vi "Convert Detection Robot to AI Robot.vi"(7 "Lado":enum16{"Esquerdo", "Direito"}(ring) caption="Enum", 11 "Input":T6[](array[typedef]) {"height" format="%+4.3f"; "pixel_y" format="%+4.3f"; "pixel_x" format="%+4.3f"; "orientation" format="%+4.3f"; "y" format="%+4.3f"; "confidence" format="%4.3f"; "x" format="%+4.3f"}) -> (3 "Output":T1[](array[typedef]))   [LabVIEW 2018]
uses:
  Controls/SSL Detection Robot.ctl
  <vilib>/Analysis/Matrix/Datatypes/RealMatrix.ctl
  Communication_class/Paths/Convert AI Robot to Robot Command Folder/Core/AI Robot.ctl
  Communication_class/Paths/Convert AI Robot to Robot Command Folder/Intel/Functions Enum.ctl
  Communication_class/Paths/Convert AI Robot to Robot Command Folder/Intel/AttackerStates.ctl
  Communication_class/Paths/Convert AI Robot to Robot Command Folder/Path Planning/RRT/PathDests.ctl
  Communication_class/Paths/Convert AI Robot to Robot Command Folder/Path Planning/RRT/PathDest.ctl
  <vilib>/Analysis/Matrix/NI_Matrix.lvlib
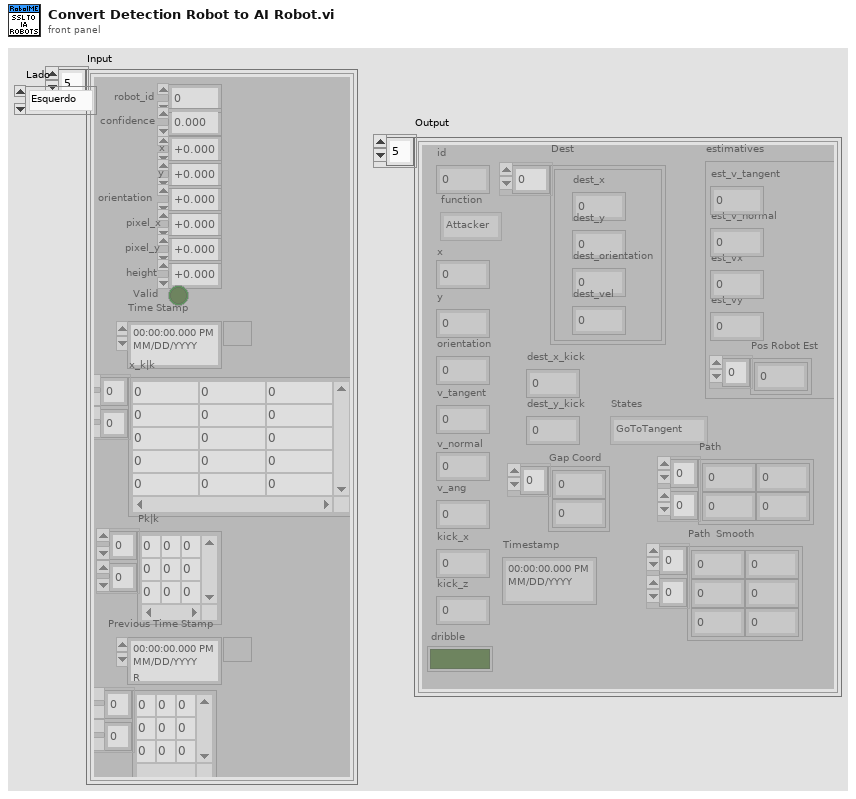
[diagram p1: front panel]
types:
  T1 = typedef "AI Robot.ctl" = cluster{"id":u32, "function":T2, "x":dbl, "y":dbl, "orientation":dbl, "v_tangent":dbl, "v_normal":dbl, "v_ang":dbl, "kick_x":dbl, "kick_z":dbl, "dribble":bool, "Timestamp":timestamp, "estimatives":cluster{"est_v_tangent":dbl, "est_v_normal":dbl, "est_vx":dbl, "est_vy":dbl, "Pos Robot Est":dbl[]}, "dest_x_kick":dbl, "dest_y_kick":dbl, "Gap Coord":dbl[], "States":T3, "Path ":dbl[][], "Path  Smooth":dbl[][], "Dest":T4}
  T2 = typedef "Functions Enum.ctl" = enum16{"2nd Striker", "Attacker", "Goalie", "Defender", "Striker", "Goto 0", "Dummy", "Kicker", "ZigZag 0", "ZigZag 1", "ZigZag 2", "ZigZag 3", "ZigZag 4", "ZigZag 5", "ZigZag 6", "ZigZag 7", "ZigZag 8", ""}
  T3 = typedef "AttackerStates.ctl" = enum16{"Pass", "GoToTangent", "BallGetting", "GoToKick", ""}
  T4 = typedef "PathDests.ctl" = T5[]
  T5 = typedef "PathDest.ctl" = cluster{"dest_x":dbl, "dest_y":dbl, "dest_orientation":dbl, "dest_vel":dbl}
  T6 = typedef "SSL Detection Robot.ctl" = cluster{"x":sgl, "robot_id":u32, "confidence":sgl, "y":sgl, "orientation":sgl, "pixel_x":sgl, "pixel_y":sgl, "height":sgl, "Valid":bool, "Time Stamp":timestamp, "x_k|k":T7, "Pk|k":T7, "Previous Time Stamp":timestamp, "R":T7}
  T7 = typedef "NI_Matrix.lvlib/RealMatrix.ctl" = dbl[][]
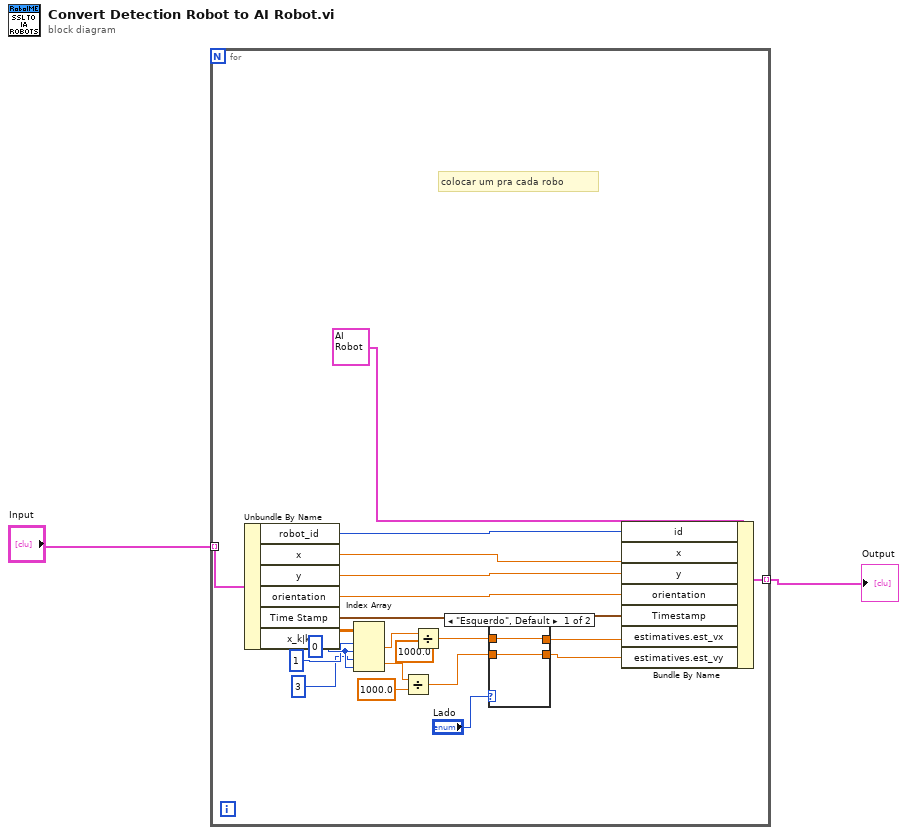
[diagram p0: block diagram]
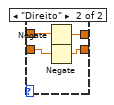
[diagram p2: hidden frame]
diagram:
  n1 = for {
    tunnel: "Input" -> [w22] mode=indexing
    tunnel: [w19] -> w1 mode=indexing
    w5 = 0 ("index (row)")
    # "colocar um pra cada robo"
    n2 = Unbundle By Name(w22) -> ("robot_id"=w8:u32, "x"=w10:sgl, "y"=w9:sgl, "orientation"=w21:sgl, "Time Stamp"=w20:timestamp, "x_k|k"=w18:T7)
    n3 = Index Array(array=w18, index (row) #1=1 ("disabled index (col)"), index (col) #1=w5, index (row) #2=3 ("index (row)"), index (col) #2=w5) -> (element #1=w17:dbl, element #2=w14:dbl)
    n4 = Divide(x=w14, y=1000.0) -> (x/y=w11:dbl)
    n5 = Divide(x=w17, y=1000.0) -> (x/y=w12:dbl)
    n6 = case shown="\"Esquerdo\", Default" "Lado" {
      tunnel: [w25 w29] -> w7
      tunnel: w12 -> [w25 w28]
      tunnel: [w24 w26] -> w6
      tunnel: w11 -> [w24 w27]
      frame "Esquerdo", Default {
      }
      frame "Direito" {
        n7 = Negate(x=w28) -> (-x=w29:dbl)
        n8 = Negate(x=w27) -> (-x=w26:dbl)
      }
    }
    n9 = Bundle By Name(cluster=T1 {"id"=0, "function"=enum."Attacker", "x"=0.0, "y"=0.0, "orientation"=0.0, "v_tangent"=0.0, "v_normal"=0.0, "v_ang"=0.0, "kick_x"=0.0, "kick_z"=0.0, "dribble"=FALSE, "Timestamp"=timestamp(0 s since 1904-01-01), "estimatives"={"est_v_tangent"=0.0, "est_v_normal"=0.0, "est_vx"=0.0, "est_vy"=0.0, "Pos Robot Est"=[]}, "dest_x_kick"=0.0, "dest_y_kick"=0.0, "Gap Coord"=[], "States"=enum."GoToTangent", "Path "=[], "Path  Smooth"=[], "Dest"=[]} ("Robot"), "id"=w8, "x"=w10, "y"=w9, "orientation"=w21, "Timestamp"=w20, "estimatives.est_vx"=w7, "estimatives.est_vy"=w6) -> (w19:T1)
  }
  "Output" <- w1
